vi "Broadcast EMIccdGainControlMode.vi"(8 "error in (no error)":errorcluster, 10 "Reply Payload":T1) -> (0 "error out":errorcluster)   [LabVIEW 2019, in "Camera.lvlib"]
doc: "_____\nCreated using Delacor QMH Event Scripter 5.0.0.112."
uses:
  Camera.lvlib
  SetGet EMIccdGainControlMode (Reply Payload)--cluster.ctl
  picam32_LabView_SDK/PICam_lib/types/PicamEMIccdGainControlMode.ctl
  picam32_LabView_SDK/PICam_lib/PICam.lvlib
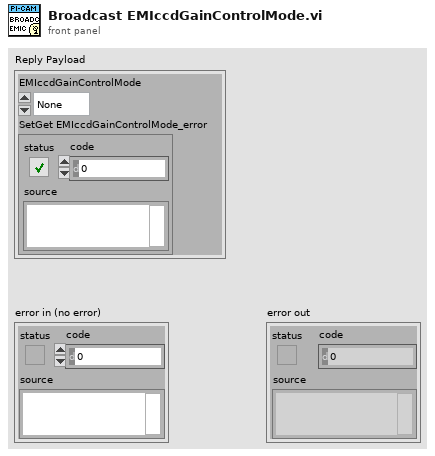
[diagram p1: front panel]
types:
  T1 = typedef "Camera.lvlib/SetGet EMIccdGainControlMode (Reply Payload)--cluster.ctl" = cluster{"EMIccdGainControlMode":T2, "SetGet EMIccdGainControlMode_error":errorcluster}
  T2 = typedef "PICam.lvlib/PicamEMIccdGainControlMode.ctl" = enum16{"None", "Optimal", "Manual"}
  T3 = typedef "Camera.lvlib/Broadcast Events--cluster.ctl" = cluster{"Module Did Init":refnum<user-event>, "Status Updated":refnum<user-event>, "Error Reported":refnum<user-event>, "Module Did Stop":refnum<user-event>, "Update Module Execution Status":refnum<user-event>, "Broadcast Image":refnum<user-event>, "Broadcast Exposure Time":refnum<user-event>, "Broadcast Binning":refnum<user-event>, "Broadcast GatingMode":refnum<user-event>, "Broadcast RepetitiveGate":refnum<user-event>, "Broadcast IntensifierStatus":refnum<user-event>, "Broadcast IntensifierGain":refnum<user-event>, "Broadcast EMIccdGainControlMode":refnum<user-event>, "Broadcast EMIccdGain":refnum<user-event>, "Broadcast FloatingPoint Parameter":refnum<user-event>, "Broadcast Integer Parameter":refnum<user-event>, "Broadcast LargeInteger Parameter":refnum<user-event>, "Broadcast Pulse Parameter":refnum<user-event>}
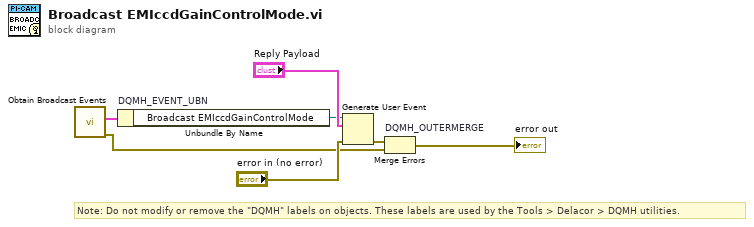
[diagram p0: block diagram]
diagram:
  # "Note: Do not modify or remove the \"DQMH\" labels on objects. These labels are used by the Tools > Delacor > DQMH utilities."
  n1 = call "Obtain Broadcast Events.vi"() -> ("error out"=w2:errorcluster, "Camera Broadcast Events"=w1:T3)  [unwired: 10 in]
  n2 = Unbundle By Name "DQMH_EVENT_UBN"(w1) -> ("Broadcast EMIccdGainControlMode"=w4:refnum<user-event>)
  n3 = Generate User Event(user event=w4, event data cluster="Reply Payload", error in="error in (no error)") -> (error out=w3:errorcluster)  [unwired: 1 in, 1 out]
  n4 = Merge Errors "DQMH_OUTERMERGE"(w3, w2) -> (→"error out":errorcluster)
